vi "Get Inertia Matrix.vi"(8 "error in (no error)":errorcluster, 11 "Link in":refnum<class "Link.lvclass">) -> (0 "error out":errorcluster, 2 "Inertia Matrix":T1, 3 "Link out":refnum<class "Link.lvclass">)   [LabVIEW 2013, in "Link.lvclass"]
uses:
  Link.lvclass
  <vilib>/Analysis/Matrix/Datatypes/RealMatrix.ctl
  Link.lvclass/Link.ctl
  <vilib>/Analysis/Matrix/NI_Matrix.lvlib
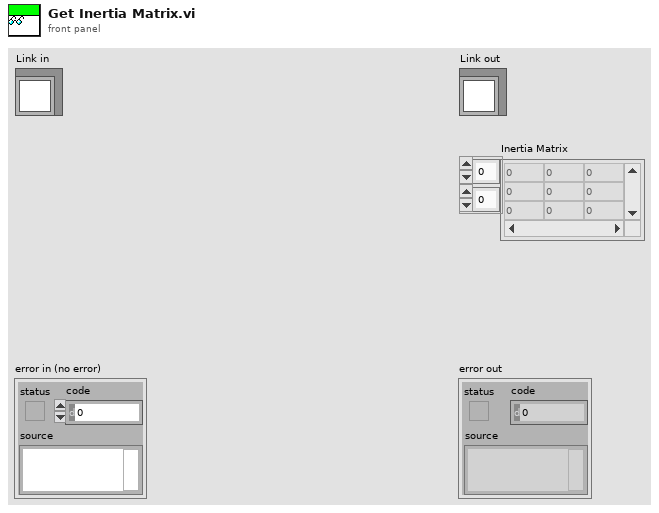
[diagram p1: front panel]
types:
  T1 = typedef "NI_Matrix.lvlib/RealMatrix.ctl" = dbl[][]
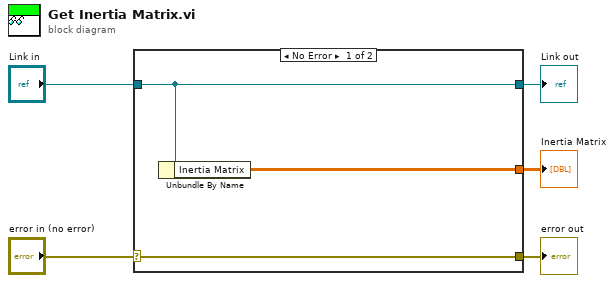
[diagram p0: block diagram]
diagram:
  n1 = case shown="No Error" "error in (no error)" {
    selector: "error in (no error)" -> [w8 w9]
    tunnel: [w8 w9] -> w4
    tunnel: [w7 w10] -> w2
    tunnel: "Link in" -> [w7 w10]
    tunnel: [w6 _] -> w1
    frame No Error {
      n2 = Unbundle By Name(w7) -> ("Inertia Matrix"=w6:T1)
    }
    frame Error {
    }
  }
  "error out" <- w4
  "Link out" <- w2
  "Inertia Matrix" <- w1
